vi "ExTestOpenCamGlobal.vi"() -> ()   [LabVIEW 2010]
uses:
  GlbCamHndls.vi
panel:
  out "error out":errorcluster
  in  "error in (no error)":errorcluster
  in  "Number of Cameras":u32=1 min=1 step=1
  # "ExTestOpenCamGlobal.vi : this sub vi opens n number of cameras \nand stores thier handles in a global variable."
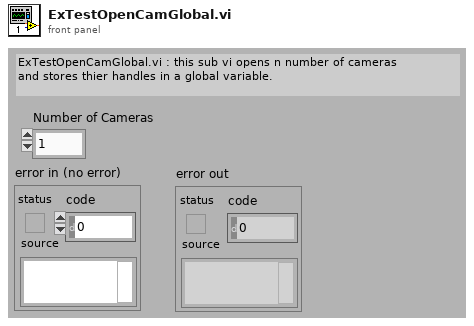
[diagram p1: front panel]
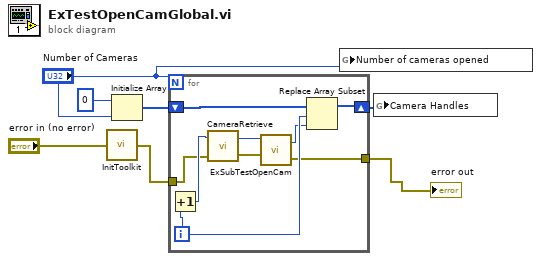
[diagram p0: block diagram]
diagram:
  n1 = call <userlib>:"InitToolkit.vi"("error in"="error in (no error)") -> ("error out"=w2:errorcluster)
  n2 = Initialize Array(0, "Number of Cameras") -> (w7:i32[])
  n3 = for {
    N: "Number of Cameras" -> [_]
    shift-right: [w12] -> w4
    shift-left: w7 -> [w14]
    tunnel: w2 -> [w8]
    tunnel: [w9] -> w1
    i -> [w16]
    n4 = Increment(x=w16) -> (x+1=w15:i32)
    n5 = call <userlib>:"CameraRetrieve.vi"("error in"=w8, "Camera Index"=w15) -> ("error out"=w10:errorcluster, "Device ID"=w13:u32)
    n6 = call "ExSubTestOpenCam.vi"("error in (no error)"=w10, "Camera Device ID"=w13) -> ("error out"=w9:errorcluster, "Camera Handle"=w11:u32)
    n7 = Replace Array Subset(array=w14, new element=w11, index=w16) -> (w12:i32[])
  }
  "error out" <- w1
  n8 = global write "GlbCamHndls.vi" "Number of cameras opened"("Number of Cameras") -> ()
  n9 = global write "GlbCamHndls.vi" "Camera Handles"(w4) -> ()
